vi "Get XY Cluster.vi"(11 "Point.lvclass":refnum<class "Point.lvclass">) -> (3 "XY Cluster":cluster{"X":i16, "Y":i16})   [LabVIEW 2017, in "Point.lvclass"]
doc: "Get the X and Y coordinates of the point."
uses:
  Point.lvclass
  Point.lvclass/Point.ctl
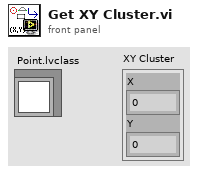
[diagram p1: front panel]
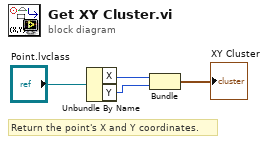
[diagram p0: block diagram]
diagram:
  # "Return the point's X and Y coordinates."
  n1 = Unbundle By Name("Point.lvclass") -> ("X"=w3:i16, "Y"=w2:i16)
  n2 = Bundle("X"=w3, "Y"=w2) -> (→"XY Cluster":cluster{"X":i16, "Y":i16})  [unwired: 1 out]
